vi "Set_Joint_Configuration_Payload.vi"(9 "Desired position":u16, 10 "Current position":u16, 11 "Identifier selection in":u8) -> (3 "Set joint position command":T1 {"payload" format="%x"; "timestamp" format="%<%I:%M:%S%8u %p\n%x>T"; "identifier" format="%x"})   [LabVIEW 2015]
uses:
  <vilib>/Stratom, Inc/X-CAN for myRIO (API)/X-CAN Class/Type Definitions/CANFrame.ctl
  <vilib>/Stratom, Inc/X-CAN for myRIO (API)/X-CAN Class/X-CAN.lvclass
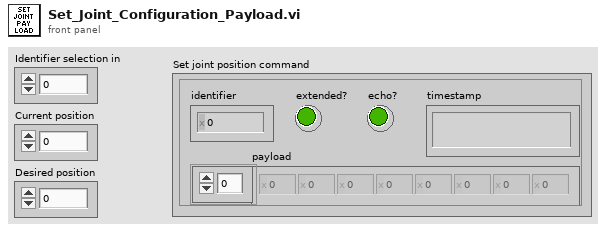
[diagram p1: front panel]
types:
  T1 = typedef "X-CAN.lvclass/CANFrame.ctl" = cluster{"identifier":u32, "extended?":bool, "echo?":bool, "payload":u8[], "timestamp":timestamp}
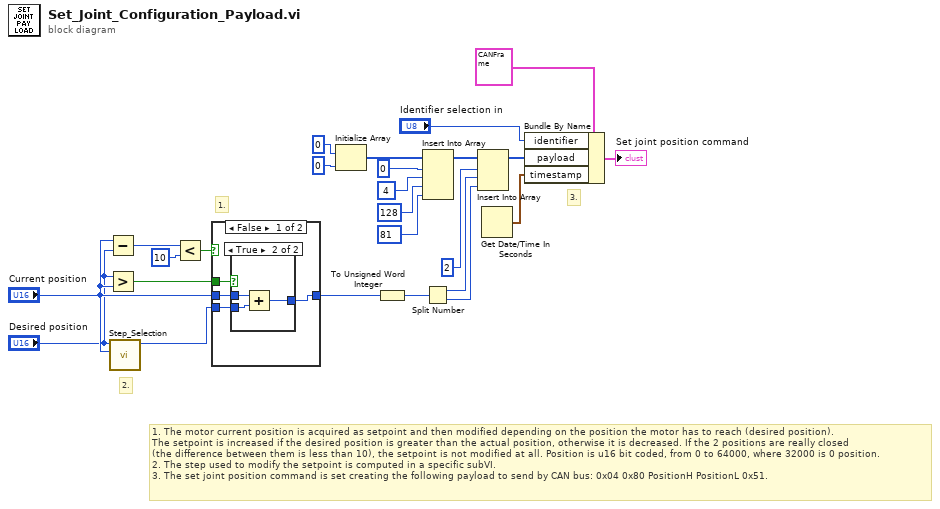
[diagram p0: block diagram]
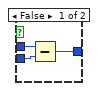
[diagram p2: hidden frame]
diagram:
  # "2."
  # "1."
  # "3."
  # "1. The motor current position is acquired as setpoint and then modified depending on the position the motor has to reach (desired position).\nThe setpoint is increased if the desired position is greater than the actual position, otherwise it is decreased. If the 2 positions are really closed\n(the difference between them is less than 10), the setpoint is not modified at all. Position is u16 bit coded, from 0 to 64000, where 32000 is 0 position.\n2. The step used to modify the setpoint is computed in a specific subVI.\n3. The set joint position command is set creating the following payload to send by CAN bus: 0x04 0x80 PositionH PositionL 0x51."
  n1 = Subtract(x="Current position", y="Desired position") -> (x-y=w6:u16)
  n2 = Greater?(x="Desired position", y="Current position") -> (0:w4:bool)
  n3 = call "Step_Selection.vi"("Current position"="Current position", "Desired position"="Desired position") -> ("Step"=w3:u16)  [unwired: 9 in]
  n4 = Less?(x=w6, y=u16 10) -> (x < y?=w8:bool)
  n5 = case shown="False" w8 {
    tunnel: [w28 w36] -> w5
    tunnel: "Current position" -> [w29 w36]
    tunnel: w4 -> [w27 _]
    tunnel: w3 -> [w26 _]
    frame False {
      n6 = case shown="True" w27 {
        tunnel: w29 -> [w32 w35]
        tunnel: [w31 w34] -> w28
        tunnel: w26 -> [w30 w33]
        frame False {
          n7 = Subtract(x=w32, y=w30) -> (x-y=w31:u16)
        }
        frame True {
          n8 = Add(x=w35, y=w33) -> (x+y=w34:u16)
        }
      }
    }
    frame True {
    }
  }
  n9 = Initialize Array(u16 0 ("element"), 0 ("dimension size")) -> (w16:u16[])
  n10 = To Unsigned Word Integer(number=w5) -> (unsigned 16bit integer=w25:u16)
  n11 = Insert Into Array(array=w16, index=0, new element #1=u8 4 ("new element/subarray"), new element #2=u8 128 ("new element/subarray"), new element #3=u8 81 ("new element/subarray")) -> (w12:u16[])
  n12 = Split Number(x=w25) -> (hi(x)=w22:u8, lo(x)=w21:u8)
  n13 = Insert Into Array(array=w12, index=2, new element #1=w22, new element #2=w21) -> (w19:u16[])
  n14 = Get Date/Time In Seconds() -> (seconds since 1Jan1904=w11:timestamp)
  n15 = Bundle By Name(cluster=T1 {"identifier"=0, "extended?"=FALSE, "echo?"=FALSE, "payload"=[], "timestamp"=timestamp(0 s since 1904-01-01)} ("CAN Frame"), "identifier"="Identifier selection in", "payload"=w19, "timestamp"=w11) -> (→"Set joint position command":T1)
